vi "run tests.vi"() -> ()   [LabVIEW 2013]
panel:
  out "Tests":T1(array[cluster])
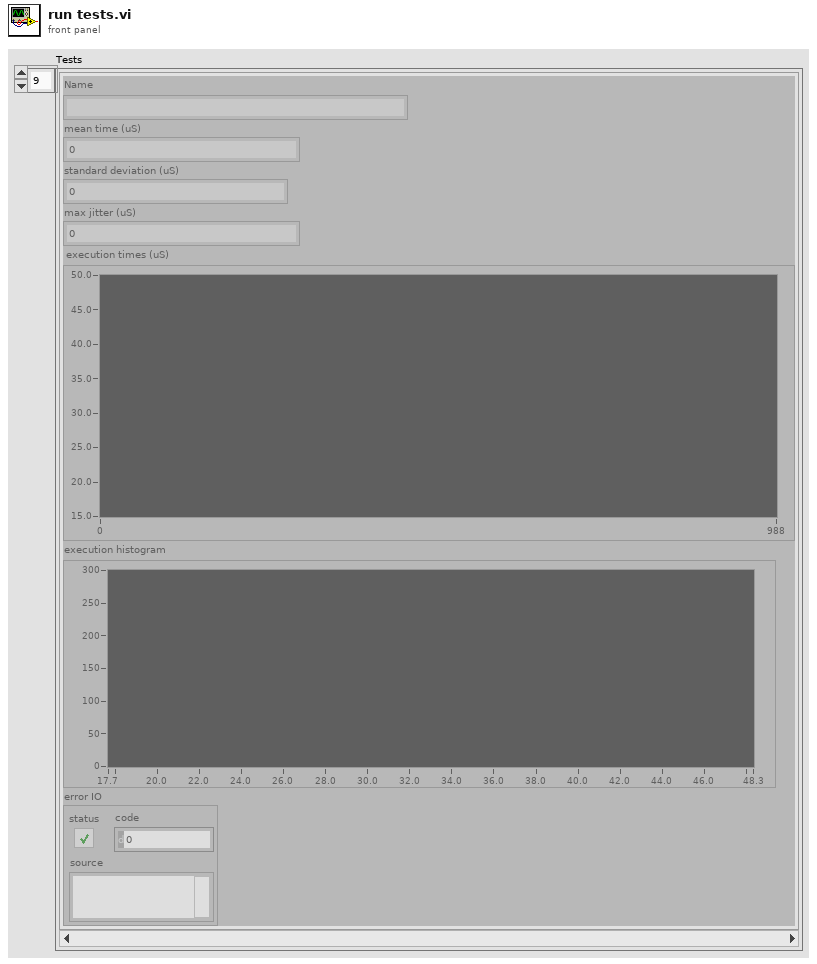
[diagram p1: front panel]
types:
  T1 = cluster{"Name":string, "mean time (uS)":dbl, "standard deviation (uS)":dbl, "max jitter (uS)":dbl, "execution times (uS)":dbl[], "execution histogram":cluster{"X Values":dbl[], "Histogram: h(x)":i32[]}, "error IO":errorcluster}[]
  T2 = cluster{"X Values":dbl[], "Histogram: h(x)":i32[]}
  T3 = cluster{"name":string, "mean time (uS)":dbl, "standard deviation (uS)":dbl, "max jitter (uS)":dbl, "execution times (uS)":dbl[], "execution histogram":cluster{"X Values":dbl[], "Histogram: h(x)":i32[]}, "error IO":errorcluster}
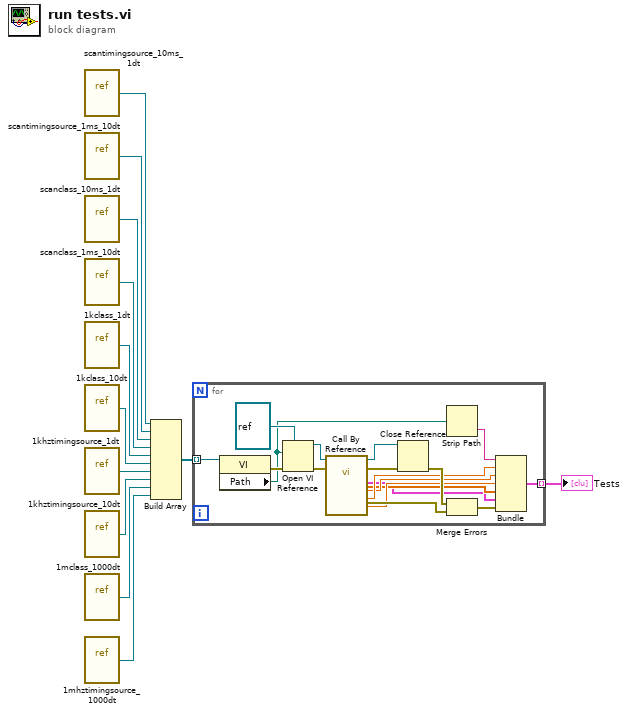
[diagram p0: block diagram]
diagram:
  n1 = vi-ref "scantimingsource_10ms_1dt.vi"() -> (w12:refnum<vi>)
  n2 = vi-ref "scantimingsource_1ms_10dt.vi"() -> (w11:refnum<vi>)
  n3 = vi-ref "scanclass_10ms_1dt.vi"() -> (w10:refnum<vi>)
  n4 = vi-ref "scanclass_1ms_10dt.vi"() -> (w9:refnum<vi>)
  n5 = vi-ref "1kclass_1dt.vi"() -> (w6:refnum<vi>)
  n6 = vi-ref "1kclass_10dt.vi"() -> (w5:refnum<vi>)
  n7 = vi-ref "1khztimingsource_1dt.vi"() -> (w4:refnum<vi>)
  n8 = vi-ref "1khztimingsource_10dt.vi"() -> (w3:refnum<vi>)
  n9 = vi-ref "1mclass_1000dt.vi"() -> (w2:refnum<vi>)
  n10 = vi-ref "1mhztimingsource_1000dt.vi"() -> (w1:refnum<vi>)
  n11 = Build Array(w12, w11, w10, w9, w6, w5, w4, w3, w2, w1) -> (w8:refnum<vi>[])
  n12 = for {
    tunnel: w8 -> [w30] mode=indexing
    tunnel: [w15] -> w7 mode=indexing
    n13 = property class="VI"(reference=w30) -> (error out=w29:errorcluster, "Path"=w14:path)  [unwired: 1 in, 1 out]
    n14 = Open VI Reference(type specifier VI Refnum (for type only)=refnum<vi> refnum, vi path=w14, error in (no error)=w29) -> (vi reference=w27:refnum<vi>, error out=w28:errorcluster)  [unwired: 3 in]
    n15 = call-by-ref "?"(reference=w27, error in=w28) -> (reference out=w24:refnum<vi>, error out=w25:errorcluster, "max jitter (uS)"=w19:dbl, "mean time (uS)"=w21:dbl, "standard deviation (uS)"=w20:dbl, "execution histogram"=w17:T2, "Error"=w22:errorcluster, "execution times (uS)"=w18:dbl[])  [unwired: 6 in]
    n16 = Close Reference(reference=w24, error in (no error)=w25) -> (error out=w23:errorcluster)
    n17 = Strip Path(path=w14) -> (name=w13:string)  [unwired: 1 out]
    n18 = Merge Errors(w23, w22) -> (w16:errorcluster)
    n19 = Bundle("name"=w13, "mean time (uS)"=w21, "standard deviation (uS)"=w20, "max jitter (uS)"=w19, "execution times (uS)"=w18, "execution histogram"=w17, "error IO"=w16) -> (w15:T3)  [unwired: 1 in]
  }
  "Tests" <- w7
